vi "Set Default VI Icon Properties.vi"(8 "error in (no error)":errorcluster, 11 "vi path":path) -> (0 "error out":errorcluster)   [LabVIEW 2020]
uses:
  <vilib>/LabVIEW Icon API/LabVIEW Icon API.lvlib
  <vilib>/LabVIEW Icon API/lv_icon/lv_icon.lvlib
  <vilib>/LabVIEW Icon API/lv_icon/Controls/Font.ctl
  <vilib>/LabVIEW Icon API/lv_icon/Controls/Alignment.ctl
  <vilib>/LabVIEW Icon API/lv_icon/Controls/BodyText.ctl
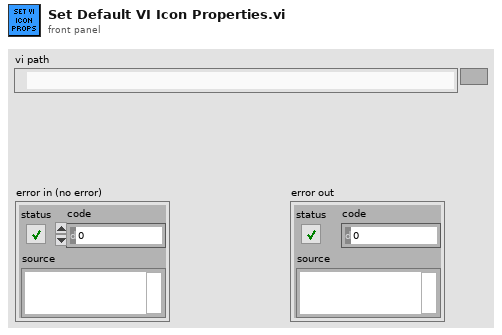
[diagram p1: front panel]
types:
  T1 = typedef "Alignment.ctl" = u16
  T2 = typedef "Font.ctl" = string
  T3 = typedef "BodyText.ctl" = cluster{"Line 1 text":string, "Line 2 text":string, "Line 3 text":string, "Line 4 text":string, "Line 1 color":u32, "Line 2 color":u32, "Line 3 color":u32, "Line 4 color":u32, "Body Text Spec":cluster{"Font":T2, "Alignment":T1, "Size":u8}, "Center text vertically":bool, "Capitalize Text":bool}
  T4 = typedef "LabVIEW Icon Stored Information.ctl" = cluster{"Text Visible?":bool, "Text Opacity":u8, "Templ Visible?":bool, "Templ Opacity":u8, "Relative Path from 1 to 2":path, "Image":picture, "All User Layers":refnum<class "Layer.lvclass">[], "Body Text":T3}
  T5 = typedef "imagedata.ctl" = cluster{"image type":i32, "image depth":i32, "image":u8[], "mask":u8[], "colors":u32[], "Rectangle":cluster{"left":i16, "top":i16, "right":i16, "bottom":i16}}
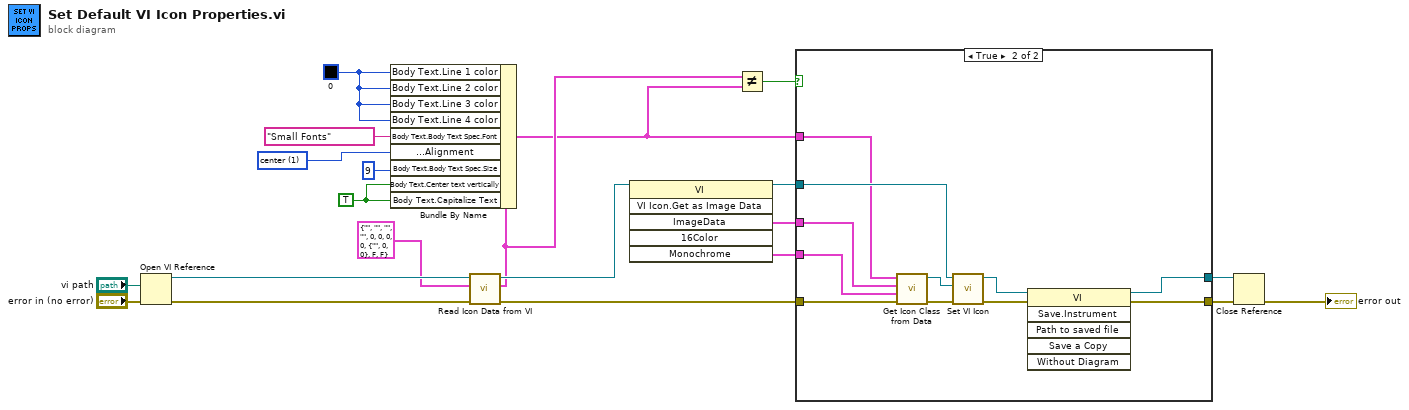
[diagram p0: block diagram]
diagram:
  w8 = T1 1 items=["left", "center", "right"] ("Body Text.Body Text Spec.Alignment")
  w10 = TRUE ("Body Text.Center text vertically")
  w11 = u32 0
  n1 = Open VI Reference(vi path="vi path", error in (no error)="error in (no error)") -> (vi reference=w21:refnum<vi>, error out=w6:errorcluster)  [unwired: 4 in]
  n2 = call <vilib>:"Read Icon Data from VI.vi"("error in (no error)"=w6, "Default body text"=T3 {"Line 1 text"="", "Line 2 text"="", "Line 3 text"="", "Line 4 text"="", "Line 1 color"=0, "Line 2 color"=0, "Line 3 color"=0, "Line 4 color"=0, "Body Text Spec"={"Font"="", "Alignment"=0, "Size"=0}, "Center text vertically"=FALSE, "Capitalize Text"=FALSE}, "VI Ref in"=w21) -> ("error out"=w20:errorcluster, "Data"=w3:T4, "VI Ref out"=w4:refnum<vi>)  [unwired: 6 in]
  n3 = Bundle By Name(cluster=w3, "Body Text.Line 1 color"=w11, "Body Text.Line 2 color"=w11, "Body Text.Line 3 color"=w11, "Body Text.Line 4 color"=w11, "Body Text.Body Text Spec.Font"=T2 "Small Fonts", "Body Text.Body Text Spec.Alignment"=w8, "Body Text.Body Text Spec.Size"=u8 9, "Body Text.Center text vertically"=w10, "Body Text.Capitalize Text"=w10) -> (w2:T4)
  n4 = invoke class="VI" method="VI Icon.Get as Image Data"(reference=w4) -> (reference out=w12:refnum<vi>, "ImageData"=w14:T5, "Monochrome"=w13:T5)  [unwired: 5 in, 3 out]
  n5 = Not Equal?(x=w3, y=w2) -> (x != y?=w1:bool)
  n6 = case shown="True" w1 {
    tunnel: w20 -> [w23 w34]
    tunnel: [w23 w33] -> w17
    tunnel: [w22 w32] -> w16
    tunnel: w14 -> [_ w31]
    tunnel: w13 -> [_ w30]
    tunnel: w12 -> [w22 w28]
    tunnel: w2 -> [_ w24]
    frame False {
    }
    frame True {
      n7 = call <vilib>:"Get Icon Class from Data.vi"("error in (no error)"=w34, "BW Icon"=w30, "Color Icon"=w31, "Icon Data"=w24) -> ("error out"=w27:errorcluster, "Icon out"=w29:refnum<class "Icon.lvclass">)  [unwired: 6 in]
      n8 = call <vilib>:"Set VI Icon.vi"("error in (no error)"=w27, "Icon"=w29, "VI Refnum in"=w28) -> ("error out"=w26:errorcluster, "VI Refnum out"=w25:refnum<vi>)  [unwired: 7 in]
      n9 = invoke class="VI" method="Save.Instrument"(reference=w25, error in=w26) -> (reference out=w32:refnum<vi>, error out=w33:errorcluster)  [unwired: 4 in, 4 out]
    }
  }
  n10 = Close Reference(reference=w16, error in (no error)=w17) -> (error out=→"error out":errorcluster)
